vi "Mutexed Merge Errors.vi"(6 "Publish Time (Use Current Time)":timestamp, 8 "error in (no error)":errorcluster, 9 "Error or Array of Errors":variant, 10 "Datum Name":string, 11 "IModel in":refnum<class "IModel.lvclass">) -> (0 "error out":errorcluster, 3 "IModel out":refnum<class "IModel.lvclass">)   [LabVIEW 2017, in "IModel.lvlib" / "IModel.lvclass"]
uses:
  <vilib>/gpm_packages/@cs/mva-core/Source/IModel/IModel/IModel.lvclass
  C:/Program Files/National Instruments/LabVIEW 2017/vi.lib/gpm_packages/@cs/mva-core/Source/IObserver/IObserver/IObserver.lvclass
  <vilib>/gpm_packages/@cs/mva-core/Source/IObserver/IObserver/IObserver.lvclass/IObserver.ctl
  <vilib>/gpm_packages/@cs/mva-core/Source/IModel/IModel/IModel.lvclass/IModel.ctl
  <vilib>/gpm_packages/@cs/mva-core/Source/PublicationPolicy/MergeErrorsPublication/MergeErrorsPublication.lvclass
  C:/Program Files/National Instruments/LabVIEW 2017/vi.lib/gpm_packages/@cs/mva-core/Source/IMediator/IPublicationPolicy/IPublicationPolicy.lvclass
  <vilib>/gpm_packages/@cs/mva-core/Source/IMediator/PublishRequest/PublishRequest.lvclass/PublishRequest.ctl
  <vilib>/gpm_packages/@cs/mva-core/Source/IMediator/MutexedPublishRequest/MutexedPublishRequest.lvclass/MutexedPublishRequest.ctl
  <vilib>/gpm_packages/@cs/mva-core/Source/IMediator/IMediator Messages/Publish Msg/Publish Msg.lvclass/Publish Msg.ctl
  <vilib>/gpm_packages/@cs/actor-framework-messages/Source/RoundTripMessage/RoundTripMessage.lvclass/RoundTripMessage.ctl
  <vilib>/ActorFramework/Message Enqueuer/Message Enqueuer.lvclass/Message Enqueuer.ctl
  <vilib>/gpm_packages/@cs/actor-framework-messages/Source/RoundTripMessage/Return Round-Trip Message.vi
  <vilib>/gpm_packages/@cs/mva-core/Source/IMediator/PublishRequest/Pack Publish Request.vi
  <vilib>/ActorFramework/Message Enqueuer/Enqueue.vi
  <vilib>/gpm_packages/@cs/mva-core/Source/IMediator/MutexedPublishRequest/MutexedPublishRequest.lvclass
  C:/Program Files/National Instruments/LabVIEW 2017/vi.lib/gpm_packages/@cs/mva-core/Source/IMediator/PublishRequest/PublishRequest.lvclass
  <vilib>/gpm_packages/@cs/mva-core/Source/IMediator/IMediator Messages/Publish Msg/Publish Msg.lvclass
  C:/Program Files/National Instruments/LabVIEW 2017/vi.lib/gpm_packages/@cs/actor-framework-messages/Source/RoundTripMessage/RoundTripMessage.lvclass
  <vilib>/gpm_packages/@cs/actor-framework-messages/Source/RoundTripMessage/RoundTripMessage.lvclass
  C:/Program Files/National Instruments/LabVIEW 2017/vi.lib/ActorFramework/Message/Message.lvclass
  <vilib>/ActorFramework/Message Priority Queue/Priority Enqueue.vi
  <vilib>/Utility/error.llb/Error Cluster From Error Code.vi
  <vilib>/gpm_packages/@cs/transport/Source/ITransport/ITransport.lvclass
  <vilib>/ErrorRing/Error Ring.xnode
  <vilib>/gpm_packages/@cs/mva-core/Source/IObserver/IObserver/IObserver.lvclass
  <vilib>/Utility/Data Type/NI_Data Type.lvlib
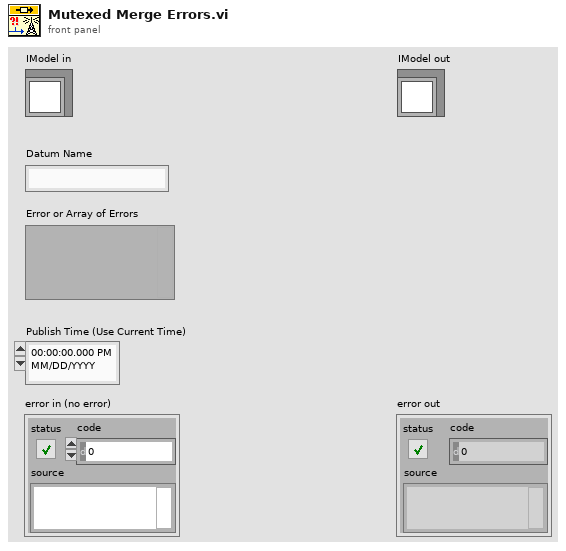
[diagram p1: front panel]
types:
  T1 = typedef "NI_Data Type.lvlib/Data Type.ctl" = enum8{"Invalid Type", "Void", "I8", "I16", "I32", "I64", "U8", "U16", "U32", "U64", "Single Float", "Double Float", "Extended Float", "Single Complex", "Double Complex", "Extended Complex", "Enum U8", "Enum U16", "Enum U32", "Enum U64", "Single Float With Unit", "Double Float With Unit", "Extended Float With Unit", "Single Complex with Unit", "Double Complex with Unit", "Extended Complex with Unit", "Boolean", "String", "Path", "Picture", "Tag", "Array", "Cluster", "Variant", "LV Variant", "Waveform", "Timestamp", "Digital Waveform", "Digital Data", "ExpressData", "Refnum", "External Data", "VI", "Poly VI", "LabVIEW Class Instance", "Fixed Point"}
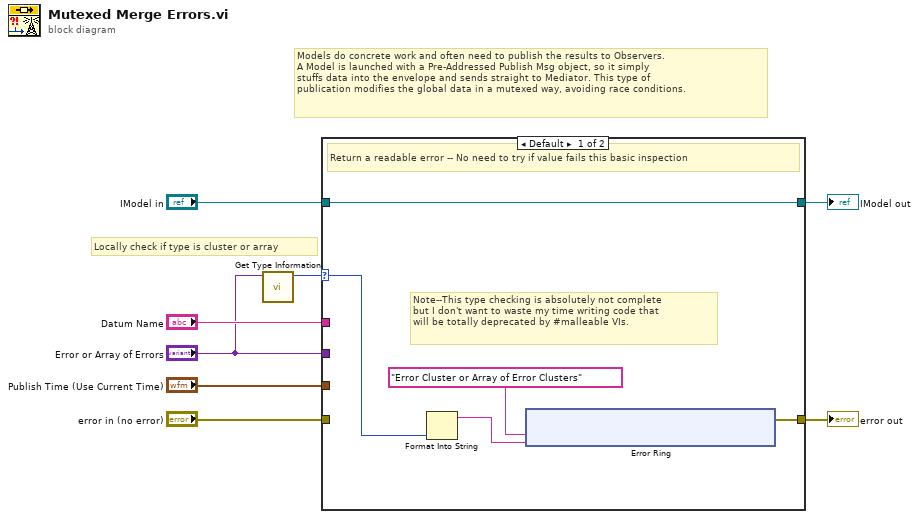
[diagram p0: block diagram]
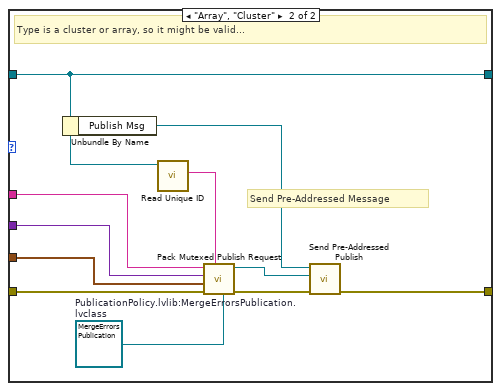
[diagram p2: hidden frame]
diagram:
  # "Locally check if type is cluster or array"
  # "Models do concrete work and often need to publish the results to Observers.\nA Model is launched with a Pre-Addressed Publish Msg object, so it simply\nstuffs data into the envelope and sends straight to Mediator. This type of\npublication modifies the global data in a mutexed way, avoiding race conditions."
  n1 = call <vilib>:"Get Type Information.vi"("Variant"="Error or Array of Errors") -> ("Type"=w1:T1)  [unwired: 6 in, 4 out]
  n2 = case shown="Default" w1 {
    selector: w1 -> [w9 _]
    tunnel: "error in (no error)" -> [_ w22]
    tunnel: [w12 w29] -> w7
    tunnel: "IModel in" -> [w13 w24]
    tunnel: "Datum Name" -> [_ w28]
    tunnel: "Error or Array of Errors" -> [_ w27]
    tunnel: "Publish Time (Use Current Time)" -> [_ w26]
    tunnel: [w13 w24] -> w3
    frame Default {
      # "Note--This type checking is absolutely not complete\nbut I don't want to waste my time writing code that\nwill be totally deprecated by #malleable VIs."
      # "Return a readable error -- No need to try if value fails this basic inspection"
      n3 = Format Into String(w9) -> (resulting string=w10:string)  [unwired: 3 in, 1 out]
      n4 = xnode "Error Ring"("parameter 0"="Error Cluster or Array of Error Clusters", "parameter 1"=w10) -> ("error out"=w12:errorcluster)
    }
    frame "Array", "Cluster" {
      w20 = refnum<class "MergeErrorsPublication.lvclass"> refnum  # PublicationPolicy.lvlib:MergeErrorsPublication.lvclass
      # "Send Pre-Addressed Message"
      # "Type is a cluster or array, so it might be valid..."
      n5 = Unbundle By Name(w24) -> ("Publish Msg"=w30:refnum<class "Publish Msg.lvclass">)
      n6 = call <vilib>:"Read Unique ID.vi"("IObserver In"=w24) -> ("Unique ID"=w23:string)  [unwired: 10 in]
      n7 = call <vilib>:"Pack Mutexed Publish Request.vi"("PublicationPolicy"=w20, "Publisher ID"=w23, "error in (no error)"=w22, "Publish Time (Use Current Time)"=w26, "Datum Value or Type"=w27, "Datum Name"=w28) -> ("error out"=w21:errorcluster, "MutexedPublishRequest Out"=w25:refnum<class "MutexedPublishRequest.lvclass">)  [unwired: 4 in]
      n8 = call <vilib>:"Send Pre-Addressed Publish.vi"("error in (no error)"=w21, "PublishRequest"=w25, "Publish Message"=w30) -> ("error out"=w29:errorcluster)  [unwired: 8 in]
    }
  }
  "IModel out" <- w3
  "error out" <- w7
